vi "AO_6738_Run_And_Stop.vi"(8 "error  in":errorcluster caption="error in", 11 "Instrument handle in":refnum<k21>) -> (0 "error out":errorcluster)   [LabVIEW 2024]
doc: "I Description: FOR TESTS PURPOSE ONLY\nThis VI inits a waveform generation session for HSDIO 6541. This is a basic example that shows how to setup the board in order to generate waveforms according to a script. \n\nII Instructions for Running:\n1. Start the VI and select any previously created sequence script.\n2. If software trigger is choosen, just click on the Send Software Trigger button to generate the sequence.\nIf not, connect an external TTL trigger to the PFI0 input pin of the HSDIO, and generation will start immediately after the next trigger pulse.\n\nIII Block Diagram Steps:\n1. Initialize for a generation session.\n2. Assign the specified channels in Channel List for dynamic operation.\n3. Configure the Sample clock to use the onboard clock, and configure the clock rate.\n\n\n\n1. Initialize for a generation session.\n2. Assign specified channels in Channel List for dynamic operation : all = \"\" (default)\n3. Sets the Idle State for when the generation has completed : NO !!\n4. Configure the Sample clock to use the onboard clock, and configure the clock rate.\n5. Set generation mode to Scripted.\n6. Configure the Script Trigger : change to Digital Edge if waiting for an external\n trigger, and link Rising Edge and source trigger commands.\n Use PFI0 with SMB wired to the board, or any PFIxx if connected to accessory.\n6. Initiate dynamic pattern generation.\n7. Wait until the generation is done.\n8. Close the generation session."
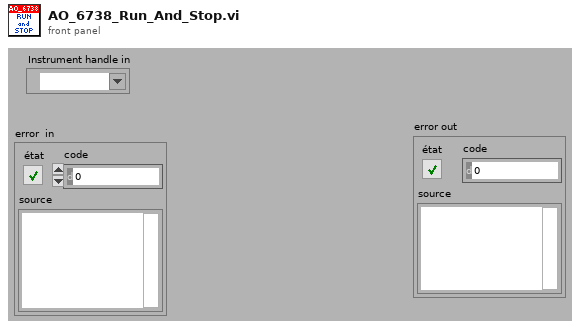
[diagram p1: front panel]
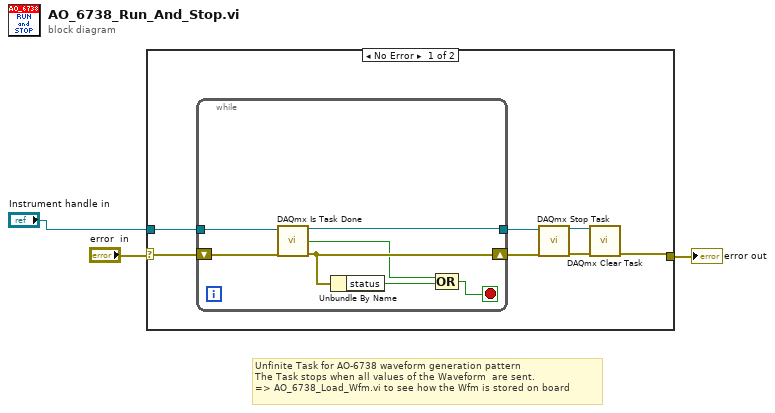
[diagram p0: block diagram]
diagram:
  # "Unfinite Task for AO-6738 waveform generation pattern\nThe Task stops when all values of the Waveform  are sent.\n=> AO_6738_Load_Wfm.vi to see how the Wfm is stored on board"
  n1 = case shown="No Error" "error  in" {
    selector: "error  in" -> [w10 w18]
    tunnel: [w6 w18] -> w3
    tunnel: "Instrument handle in" -> [w4 _]
    frame No Error {
      n2 = while {
        shift-right: [w16] -> w9
        shift-left: w10 -> [w11]
        tunnel: w4 -> [w12]
        tunnel: [w17] -> w5
        stop <- w13 stop-if-true
        n3 = call <vilib>:"DAQmx Is Task Done.vi"("task/channels in"=w12, "error in"=w11) -> ("task out"=w17:refnum<k21>, "task done?"=w15:bool, "error out"=w16:errorcluster)  [unwired: 11 in]
        n4 = Unbundle By Name(w16) -> ("status"=w14:bool)
        n5 = Compound Arithmetic op=OR ("Opérateur arithmétique")(w15, w14) -> (w13:bool)
      }
      n6 = call <vilib>:"DAQmx Stop Task.vi"("task/channels in"=w5, "error in"=w9) -> ("task out"=w8:refnum<k21>, "error out"=w7:errorcluster)  [unwired: 12 in]
      n7 = call <vilib>:"DAQmx Clear Task.vi"("task in"=w8, "error in"=w7) -> ("error out"=w6:errorcluster)  [unwired: 13 in]
    }
    frame Error {
    }
  }
  "error out" <- w3
